vi "Set Safe State.vi"(8 "error in":errorcluster, 9 "timeout (-1)":i32=-1, 11 "Standard Engine Runtime in":refnum<class "Standard Engine Runtime.lvclass">) -> (0 "error out":errorcluster, 3 "Standard Engine Runtime out":refnum<class "Standard Engine Runtime.lvclass">)   [LabVIEW 2013, in "Standard Engine Runtime.lvclass"]
doc: "This method commands the engine to enter its configured safe-state."
uses:
  Standard Engine Runtime.lvclass
  engine state.ctl
  Standard Engine Runtime.lvclass/Standard Engine Runtime.ctl
  main engine/main engine.lvlib
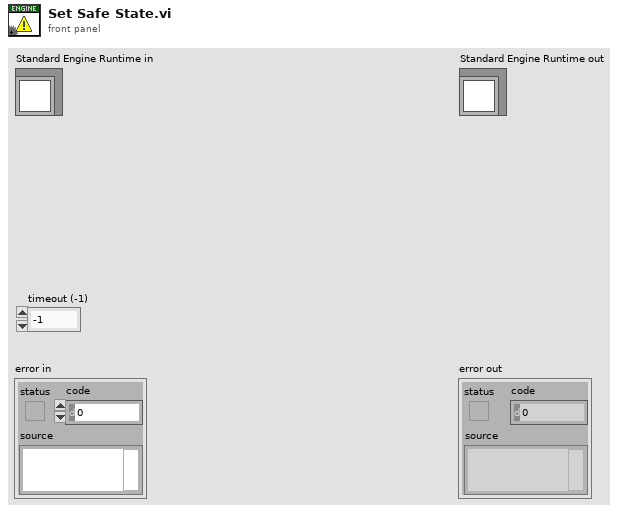
[diagram p1: front panel]
types:
  T1 = typedef "main engine.lvlib/engine state.ctl" = enum16{"idle", "configured", "running", "safe state", "exit"}
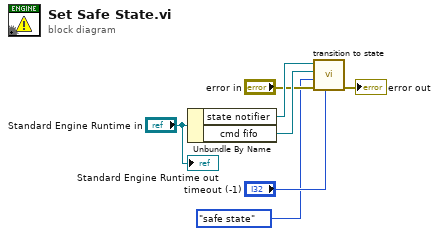
[diagram p0: block diagram]
diagram:
  n1 = Unbundle By Name("Standard Engine Runtime in") -> ("state notifier"=w6:refnum<notifier>, "cmd fifo"=w5:refnum<k33>)
  n2 = call "transition to state.vi"("timeout"="timeout (-1)", "error in"="error in", "state"=engine_state."safe state", "cmd fifo"=w5, "notifier"=w6) -> ("error out"=→"error out":errorcluster)  [unwired: 6 in]
  "Standard Engine Runtime out" <- "Standard Engine Runtime in"
